vi "Read FolderName (Row).vi"(8 "error in (no error)":errorcluster, 11 "Folder_Mgmt in":refnum<class "Folder_Mgmt.lvclass">) -> (0 "error out":errorcluster, 2 "FolderName (Row)":string[](array[string]), 3 "Folder_Mgmt out":refnum<class "Folder_Mgmt.lvclass">)   [LabVIEW 2016, in "Folder_Mgmt.lvclass"]
uses:
  Folder_Mgmt.lvclass
  Folder_Mgmt.lvclass/Folder_Mgmt.ctl
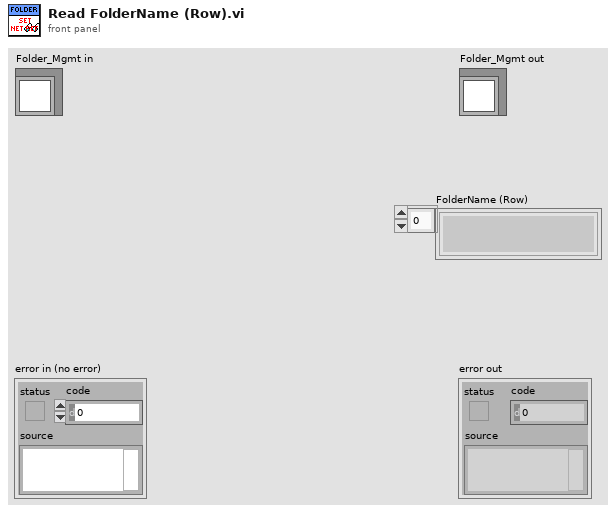
[diagram p1: front panel]
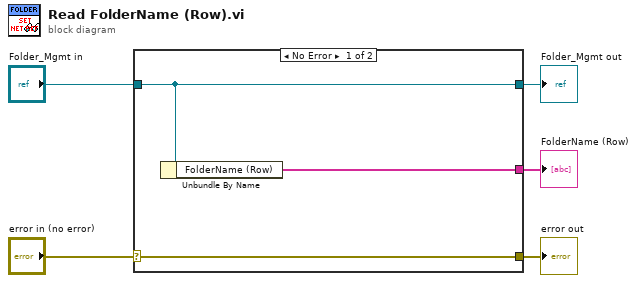
[diagram p0: block diagram]
diagram:
  n1 = case shown="No Error" "error in (no error)" {
    selector: "error in (no error)" -> [w8 w9]
    tunnel: [w8 w9] -> w4
    tunnel: [w7 w10] -> w2
    tunnel: "Folder_Mgmt in" -> [w7 w10]
    tunnel: [w6 _] -> w1
    frame No Error {
      n2 = Unbundle By Name(w7) -> ("FolderName (Row)"=w6:string[])
    }
    frame Error {
    }
  }
  "error out" <- w4
  "Folder_Mgmt out" <- w2
  "FolderName (Row)" <- w1
